vi "Initialize.vi"(8 "error in (no error)":errorcluster, 11 "DAQ_QPT_Throlab in":refnum<class "DAQ_QPT_Throlab.lvclass">) -> (0 "error out":errorcluster, 3 "DAQ_QPT_Throlab out":refnum<class "DAQ_QPT_Throlab.lvclass">)   [LabVIEW 2020, in "DAQ_QPT_Throlab.lvlib" / "DAQ_QPT_Throlab.lvclass"]
uses:
  DAQ_QPT_Throlab.lvclass
  DAQ_QPT_Throlab.lvclass/DAQ_QPT_Throlab.ctl
  Hardware Abstraction Layer/Component/DAQ/DAQ/DAQ.lvclass
  Dependency/TIRF-Lock.dll
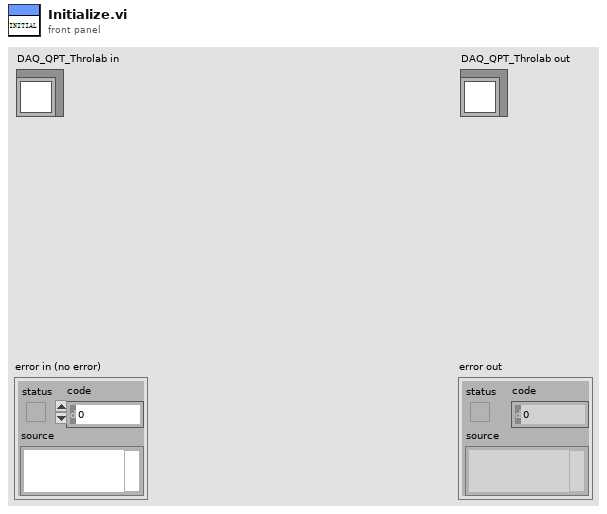
[diagram p1: front panel]
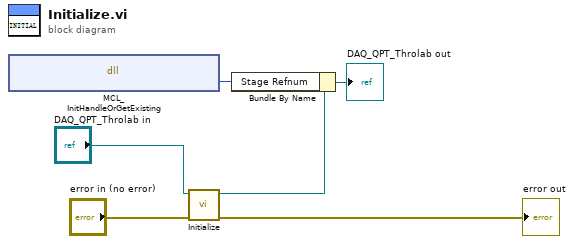
[diagram p0: block diagram]
diagram:
  n1 = dll-call lib="E:/Development/DevHardSoftware/MicroscopyFramework/Model/Hardware Layer/Real Hardware/DAQ_QPT_Throlab/DAQ_QPT_Throlab/Dependency/TIRF-Lock.dll" fn="MCL_InitHandleOrGetExisting" label="TIRF handle"() -> ("handle"=w4:i32)  [unwired: 3 in, 2 out]
  n2 = call-parent "Initialize.vi"("error in (no error)"="error in (no error)", "DAQ in"="DAQ_QPT_Throlab in") -> ("error out"=→"error out":errorcluster, "DAQ out"=w2:refnum<class "DAQ_QPT_Throlab.lvclass">)  [unwired: 8 in]
  n3 = Bundle By Name(cluster=w2, "Stage Refnum"=w4) -> (→"DAQ_QPT_Throlab out":refnum<class "DAQ_QPT_Throlab.lvclass">)
